vi "Identify and Replace Element Attribute.vi"(7 "Replacement Attribute Type":string, 8 "Identifying Attribute Value":string, 9 "Identifying Attribute Type":string, 10 "Element Type":string, 11 "XML String":string) -> (3 "Edited XML":string)   [LabVIEW 2019, in "EditSVG.lvclass"]
uses:
  EditSVG.lvclass
panel:
  in  "Replacement Attribute Value":string
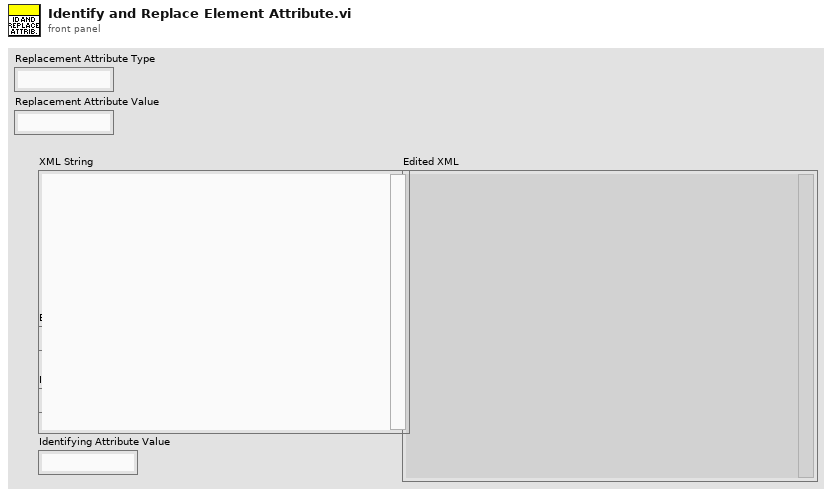
[diagram p1: front panel]
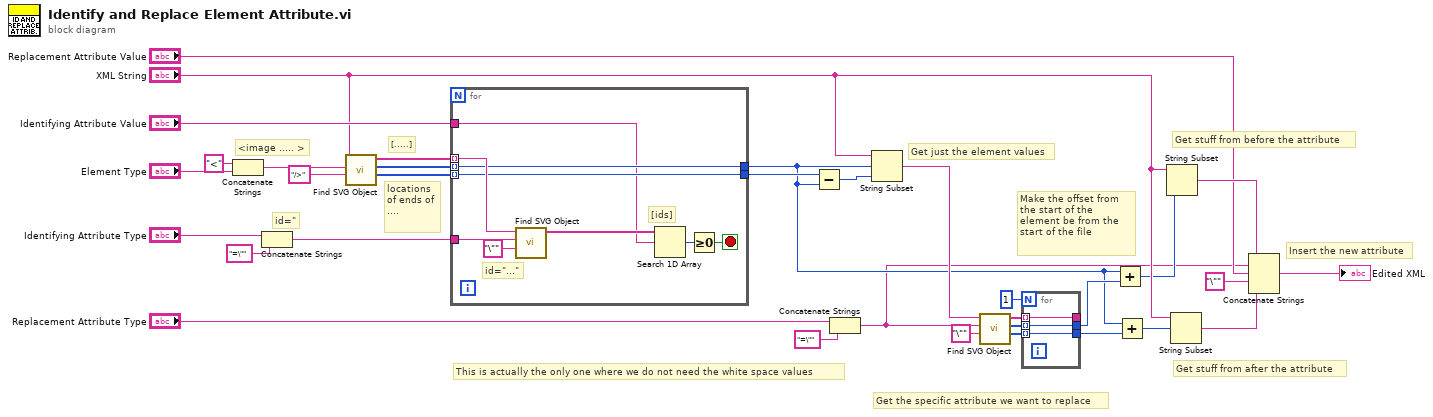
[diagram p0: block diagram]
diagram:
  # "This is actually the only one where we do not need the white space values"
  # "Get stuff from after the attribute"
  # "Get stuff from before the attribute"
  # "Insert the new attribute"
  # "Make the offset from the start of the element be from the start of the file"
  # "Get the specific attribute we want to replace"
  # "Get just the element values"
  # "id=\""
  # "locations of ends of ...."
  # "[.....]"
  # "<image ..... >"
  n1 = Concatenate Strings("<" ("string"), "Element Type") -> (w27:string)
  n2 = Concatenate Strings("Identifying Attribute Type", "=\"" ("string")) -> (w30:string)
  n3 = call "Find SVG Object.vi"("Ending Delimiter"="/>", "Beginning Delimiter"=w27, "XML String"="XML String") -> ("Ending Indices"=w29:i32[], "Beginning Indices"=w23:i32[], "Found Values"=w32:string[])  [unwired: 6 in]
  n4 = for {
    tunnel: w32 -> [w42] mode=indexing
    tunnel: w30 -> [w40]
    tunnel: "Identifying Attribute Value" -> [w34]
    tunnel: w29 -> [w39] mode=indexing
    tunnel: [w39] -> w22
    tunnel: [w35] -> w12
    tunnel: w23 -> [w35] mode=indexing
    stop <- w36 stop-if-true
    # "id=\"...\""
    # "[ids]"
    n5 = call "Find SVG Object.vi"("Ending Delimiter"="\"", "Beginning Delimiter"=w40, "XML String"=w42) -> ("Found Values"=w38:string[])  [unwired: 6 in, 2 out]
    n6 = Search 1D Array(1D array=w38, element=w34) -> (index of element=w37:i32)  [unwired: 1 in]
    n7 = Greater Or Equal To 0?(x=w37) -> (x >= 0?=w36:bool)
  }
  n8 = Subtract(x=w22, y=w12) -> (x-y=w21:i32)
  n9 = Concatenate Strings("Replacement Attribute Type", "=\"" ("string")) -> (w4:string)
  n10 = String Subset(string="XML String", offset (0)=w12, length (rest)=w21) -> (substring=w20:string)
  n11 = call "Find SVG Object.vi"("Ending Delimiter"="\"", "Beginning Delimiter"=w4, "XML String"=w20) -> ("Ending Indices"=w14:i32[], "Beginning Indices"=w15:i32[], "Found Values"=w16:string[])  [unwired: 6 in]
  n12 = for {
    N: 1 -> [_]
    tunnel: w16 -> [w45] mode=indexing
    tunnel: [w45] -> _
    tunnel: [w44] -> w13
    tunnel: w15 -> [w44] mode=indexing
    tunnel: [w43] -> w11
    tunnel: w14 -> [w43] mode=indexing
  }
  n13 = Add(x=w12, y=w13) -> (x+y=w8:i32)
  n14 = Add(x=w12, y=w11) -> (x+y=w9:i32)
  n15 = String Subset(string="XML String", length (rest)=w8) -> (substring=w6:string)  [unwired: 1 in]
  n16 = String Subset(string="XML String", offset (0)=w9) -> (substring=w7:string)  [unwired: 1 in]
  n17 = Concatenate Strings(w6, w4, "Replacement Attribute Value", "\"" ("string"), w7) -> (→"Edited XML":string)
